vi "MCListbox Check Empty Cells.vi"(8 "Error In":errorcluster, 11 "MulticolumnListbox in":refnum<vi>) -> (0 "Error Out":errorcluster, 1 "Edit Position Now":T1, 2 "No Empty Cells (except for last row)":bool, 3 "MulticolumnListbox out":refnum<vi>, 4 "Empty Columns?":i32[](array[numeric]), 6 "last row":i32)   [LabVIEW 2013]
uses:
  <vilib>/Utility/miscctls.llb/LVRowAndColumnTypeDef.ctl
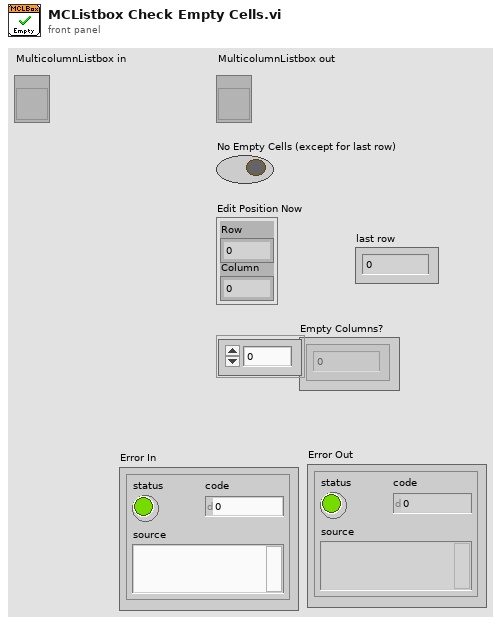
[diagram p1: front panel]
types:
  T1 = typedef "LVRowAndColumnTypeDef.ctl" = cluster{"Row":i32, "Column":i32}
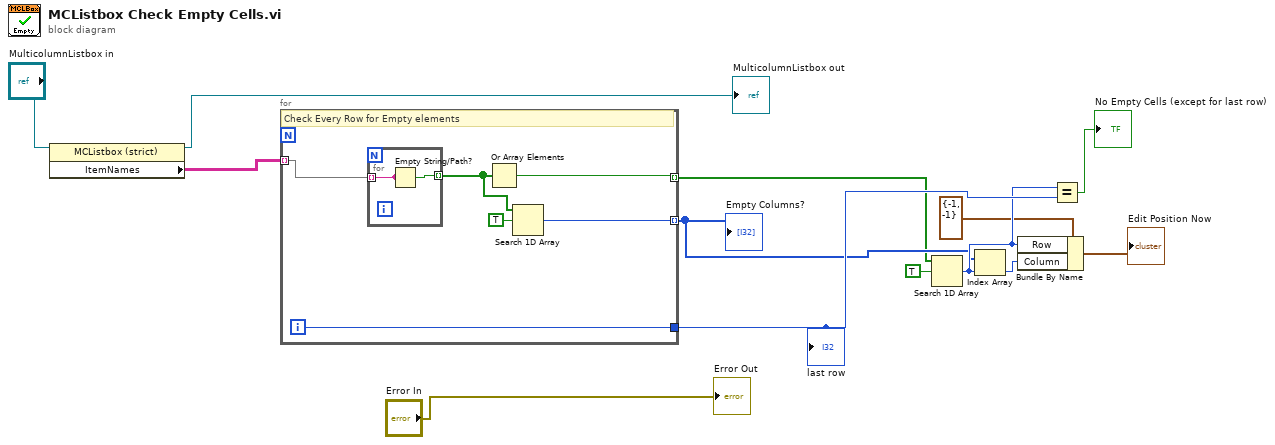
[diagram p0: block diagram]
diagram:
  n1 = property class="MCListbox (strict)"(reference="MulticolumnListbox in") -> (reference out=→"MulticolumnListbox out":refnum<vi>, "ItemNames"=w3:string[][])  [unwired: 1 in, 1 out]
  n2 = for {
    tunnel: w3 -> [w14] mode=indexing
    tunnel: [w17] -> w4 mode=indexing
    tunnel: [w16] -> w5 mode=indexing
    tunnel: [w15] -> w10
    i -> [w15]
    # "Check Every Row for Empty elements"
    n3 = for {
      tunnel: w14 -> [w21] mode=indexing
      tunnel: [w21] -> _ mode=indexing
      tunnel: [w20] -> w18 mode=indexing
      n4 = Empty String/Path?(string/path=w21) -> (empty?=w20:bool)
    }
    n5 = Or Array Elements(Boolean array=w18) -> (logical OR=w17:bool)
    n6 = Search 1D Array(1D array=w18, element=TRUE) -> (index of element=w16:i32)  [unwired: 1 in]
  }
  "Empty Columns?" <- w5
  "last row" <- w10
  n7 = Search 1D Array(1D array=w4, element=TRUE) -> (index of element=w9:i32)  [unwired: 1 in]
  n8 = Index Array(array=w5, index=w9) -> (element=w7:i32)
  n9 = Bundle By Name(cluster=T1 {"Row"=-1, "Column"=-1} ("Edit Position Now"), "Row"=w9, "Column"=w7) -> (→"Edit Position Now":T1)
  n10 = Equal?(x=w9, y=w10) -> (x = y?=→"No Empty Cells (except for last row)":bool)
  "Error Out" <- "Error In"
